vi "CLSUIP_OverrideAuthentication.vi"(8 "error in (no error)":errorcluster, 11 "VIRetooler":refnum<class "VIRetooler.lvclass">) -> (0 "error out":errorcluster, 2 "Cancelled?":bool)   [LabVIEW 2021, in "MemberVICreation.lvlib" / "VIRetooler.lvclass"]
uses:
  <resource>/Framework/Providers/LVClassLibrary/NewAccessors/VIRetooler/VIRetooler.lvclass
panel:
  in  "Incorrect Pwd":string="Incorrect password"
  out "prompt":string="%s is password-protected.  You must enter the password to create a VI for override using this VI as a template."
  in  "Cancel":bool
  in  "Verify":bool
  in  "Password":string
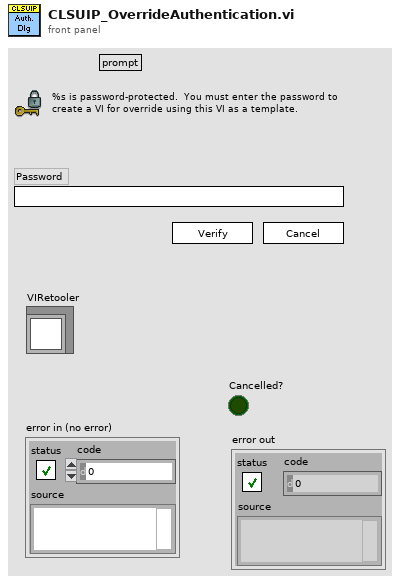
[diagram p1: front panel]
types:
  T1 = enum32{"invalid lock state", "Not Locked", "Locked (No Password)", "Password-protected"}
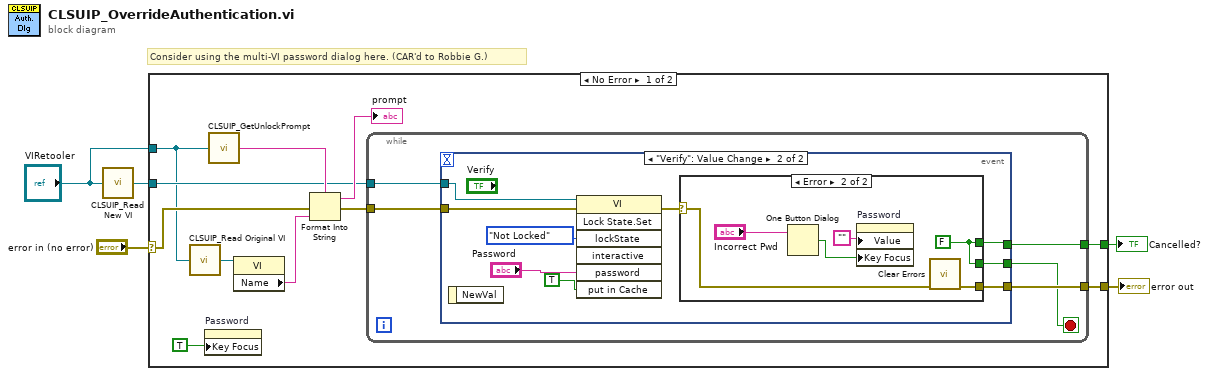
[diagram p0: block diagram]
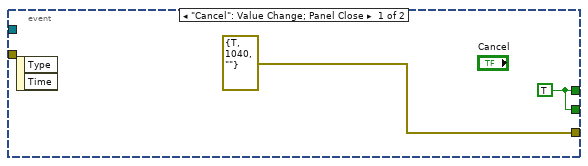
[diagram p2: hidden frame]
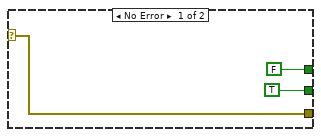
[diagram p3: hidden frame]
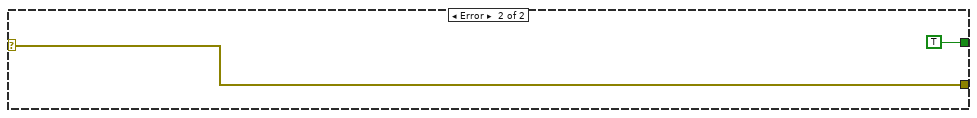
[diagram p4: hidden frame]
diagram:
  # "Consider using the multi-VI password dialog here. (CAR'd to Robbie G.)"
  n1 = call <resource>:"CLSUIP_Read New VI.vi"("VIRetooler.lvclass in"="VIRetooler") -> ("New VI"=w2:refnum<vi>)
  n2 = case shown="No Error" "error in (no error)" {
    selector: "error in (no error)" -> [w11 w43]
    tunnel: [w16 TRUE ("Put in Cache")] -> w5
    tunnel: w2 -> [w10 _]
    tunnel: [w15 w43] -> w4
    tunnel: "VIRetooler" -> [w8 _]
    frame No Error {
      n3 = call <resource>:"CLSUIP_Read Original VI.vi"("VIRetooler.lvclass in"=w8) -> ("Original VI"=w7:refnum<vi>)
      n4 = property on="Password" class="Str"("Key Focus"=TRUE) -> ()  [unwired: 2 in, 2 out]
      n5 = call-dynamic "CLSUIP_GetUnlockPrompt.vi"("VIRetooler"=w8) -> ("localized prompt 2"=w14:string)
      n6 = property class="VI"(reference=w7) -> ("Name"=w6:string)  [unwired: 1 in, 2 out]
      n7 = Format Into String(format string=w14, error in=w11, w6) -> (resulting string=→"prompt":string, error out=w12:errorcluster)  [unwired: 1 in]
      n8 = while {
        tunnel: [w18] -> w16
        tunnel: w10 -> [w21]
        tunnel: [w20] -> w15
        tunnel: w12 -> [w19]
        stop <- w17 stop-if-true
        n9 = event shown="[1] \"Verify\": Value Change" {
          selector: _ -> [_ _]
          dyn-events: _ -> [_ _]
          timeout: _ -> [_ _]
          tunnel: [w22 w27] -> w18
          tunnel: w21 -> [_ w32]
          tunnel: [errorcluster {"status"=TRUE, "code"=1040, "source"=""} ("error out") w28] -> w20
          tunnel: w19 -> [_ w26]
          tunnel: [w22 w25] -> w17
          event "Cancel": Value Change; Panel Close {
            w22 = TRUE ("Put in Cache")
            n10 = event-data() -> ()  [unwired: 3 out]
          }
          event "Verify": Value Change {
            n11 = event-data() -> ()  [unwired: 2 out]
            n12 = invoke class="VI" method="Lock State.Set"(reference=w32, error in=w26, "lockState"=T1."Not Locked" ("Lock State"), "password"="Password", "put in Cache"=TRUE ("Put in Cache")) -> (error out=w29:errorcluster)  [unwired: 2 in, 6 out]
            n13 = case shown="Error" w29 {
              selector: w29 -> [w35 w39]
              tunnel: [w35 w40] -> w28
              tunnel: [FALSE ("Put in Cache") w36] -> w27
              tunnel: [TRUE ("Put in Cache") w36] -> w25
              frame No Error {
              }
              frame Error {
                w36 = FALSE ("Put in Cache")
                n14 = One Button Dialog(message="Incorrect Pwd") -> (true=w38:bool)  [unwired: 1 out]
                n15 = property on="Password" class="Str"("Value"="", "Key Focus"=w38) -> ()  [unwired: 2 in, 2 out]
                n16 = call <vilib>:"Clear Errors.vi"("error in (no error)"=w39) -> ("error out"=w40:errorcluster)  [unwired: 1 in, 5 out]
              }
            }
          }
        }
      }
    }
    frame Error {
    }
  }
  "Cancelled?" <- w5
  "error out" <- w4
